vi "Get Pointer From Label.vi"(10 "Label":string, 11 "Offset":i32) -> (2 "Absolut Pointer":u32, 3 "Relative Pointer":u32)   [LabVIEW 2021, in "FakedArray.lvclass"]
uses:
  <resource>/plugins/NIIconEditor/Class/FakedArray/FakedArray.lvclass
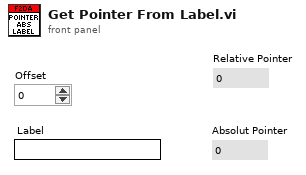
[diagram p1: front panel]
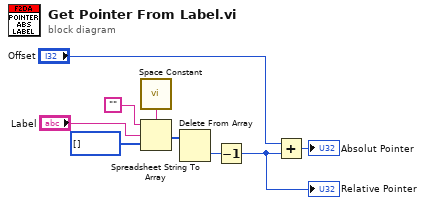
[diagram p0: block diagram]
diagram:
  n1 = call <vilib>:"Space Constant.vi"() -> ("String"=w3:string)
  n2 = Spreadsheet String To Array(delimiter (Tab)=w3, format string="", spreadsheet string="Label", array type (2D Dbl)=u32[] []) -> (array=w5:u32[])
  n3 = Delete From Array(array=w5) -> (deleted portion=w6:u32)  [unwired: 2 in, 1 out]
  n4 = Decrement(x=w6) -> (x-1=w1:u32)
  "Relative Pointer" <- w1
  n5 = Add(x="Offset", y=w1) -> (x+y=→"Absolut Pointer":u32)
